vi "Update Room Size.vi"(0 "Guest Manager UI in":refnum<class "Guest Manager UI.lvclass">, 5 "Room Sizes":string[](array[string]), 11 "error in (no error)":errorcluster) -> (4 "Guest Manager UI out":refnum<class "Guest Manager UI.lvclass">, 15 "error out":errorcluster)   [LabVIEW 2023, in "Guest Manager UI.lvlib" / "Guest Manager UI.lvclass"]
uses:
  Guest Manager UI.lvclass
  Guest Manager UI.lvclass/Guest Manager UI.ctl
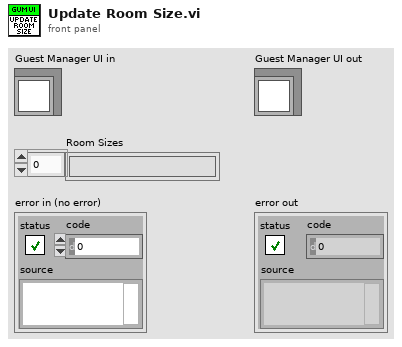
[diagram p1: front panel]
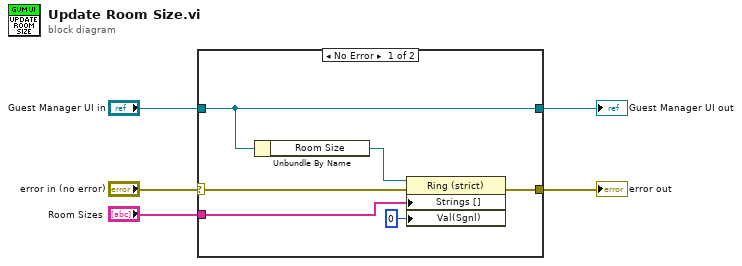
[diagram p0: block diagram]
diagram:
  n1 = case shown="No Error" "error in (no error)" {
    selector: "error in (no error)" -> [w11 w13]
    tunnel: [w10 w13] -> w4
    tunnel: [w9 w12] -> w2
    tunnel: "Guest Manager UI in" -> [w9 w12]
    tunnel: "Room Sizes" -> [w7 _]
    frame No Error {
      n2 = Unbundle By Name(w9) -> ("Room Size"=w8:refnum<vi>)
      n3 = property class="Ring (strict)"(reference=w8, error in=w11, "Strings []"=w7, "Val(Sgnl)"=u16 0 ("Value (Signaling)")) -> (error out=w10:errorcluster)  [unwired: 1 out]
    }
    frame Error {
    }
  }
  "error out" <- w4
  "Guest Manager UI out" <- w2
